vi "6AxisAccelGyro.vi"() -> ()   [LabVIEW 2024]
uses:
  Driver/Public/Digital Pull Direction.ctl
  Register.ctl
  51c12f6e-4a21-4d98-9fb3-1a2e6b8270e3.vi
  Driver/CTIPicoVISA.lvlib
panel:
  out "Waveform Chart":cluster{"[0]":dbl, "[1]":dbl, "[2]":dbl}(graph)
  out "Array":dbl[](array[numeric]) format="%.2f"
  out "loop":i32
  out "Identity":T1
  in  "Grove Connector":enum16{"I2C0", "I2C1"}(ring)
  in  "stop":bool
  in  "VISA resource name in":refnum<visa-resource-name>="COM7"
  out "error out":errorcluster
  # "https://wiki.seeedstudio.com/Grove-6-Axis_AccelerometerAndGyroscope/"
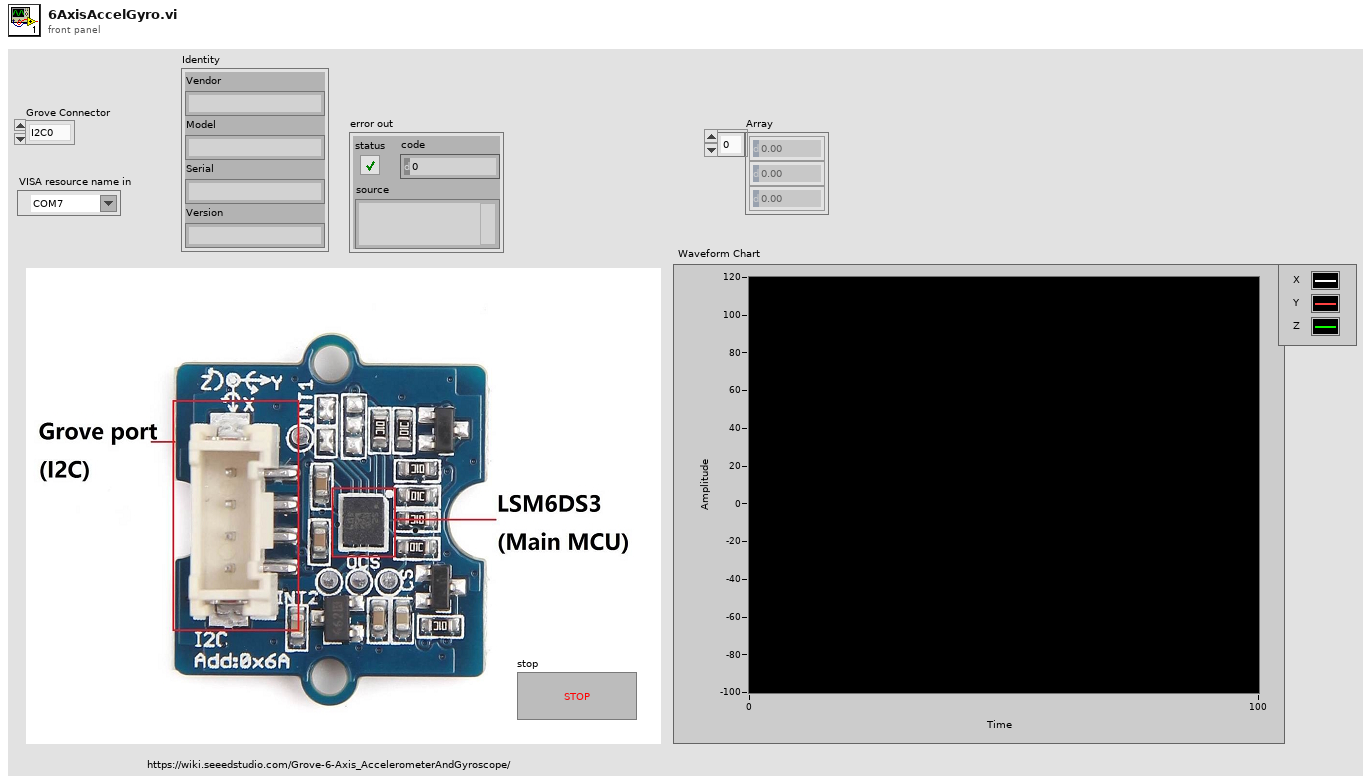
[diagram p1: front panel]
types:
  T1 = cluster{"Vendor":string, "Model":string, "Serial":string, "Version":string}
  T2 = typedef "CTIPicoVISA.lvlib/Digital Pull Direction.ctl" = enum16{"None", "Up", "Down", "Both"}
  T3 = typedef "Register.ctl" = enum16{"No Register - Error", "D6D_SRC", "STATUS_REG", "OUT_TEMP_L", "OUT_TEMP_H", "OUTX_L_G", "OUTX_H_G", "OUTY_L_G", "OUTY_H_G", "OUTZ_L_G", "OUTZ_H_G", "OUTX_L_XL", "OUTX_H_XL", "OUTY_L_XL", "OUTY_H_XL", "OUTZ_L_XL", "OUTZ_H_XL", "SENSORHUB1_REG", "SENSORHUB2_REG", "SENSORHUB3_REG", "SENSORHUB4_REG", "SENSORHUB5_REG", "SENSORHUB6_REG", "SENSORHUB7_REG", "SENSORHUB8_REG", "SENSORHUB9_REG", "SENSORHUB10_REG", "SENSORHUB11_REG", "SENSORHUB12_REG"}
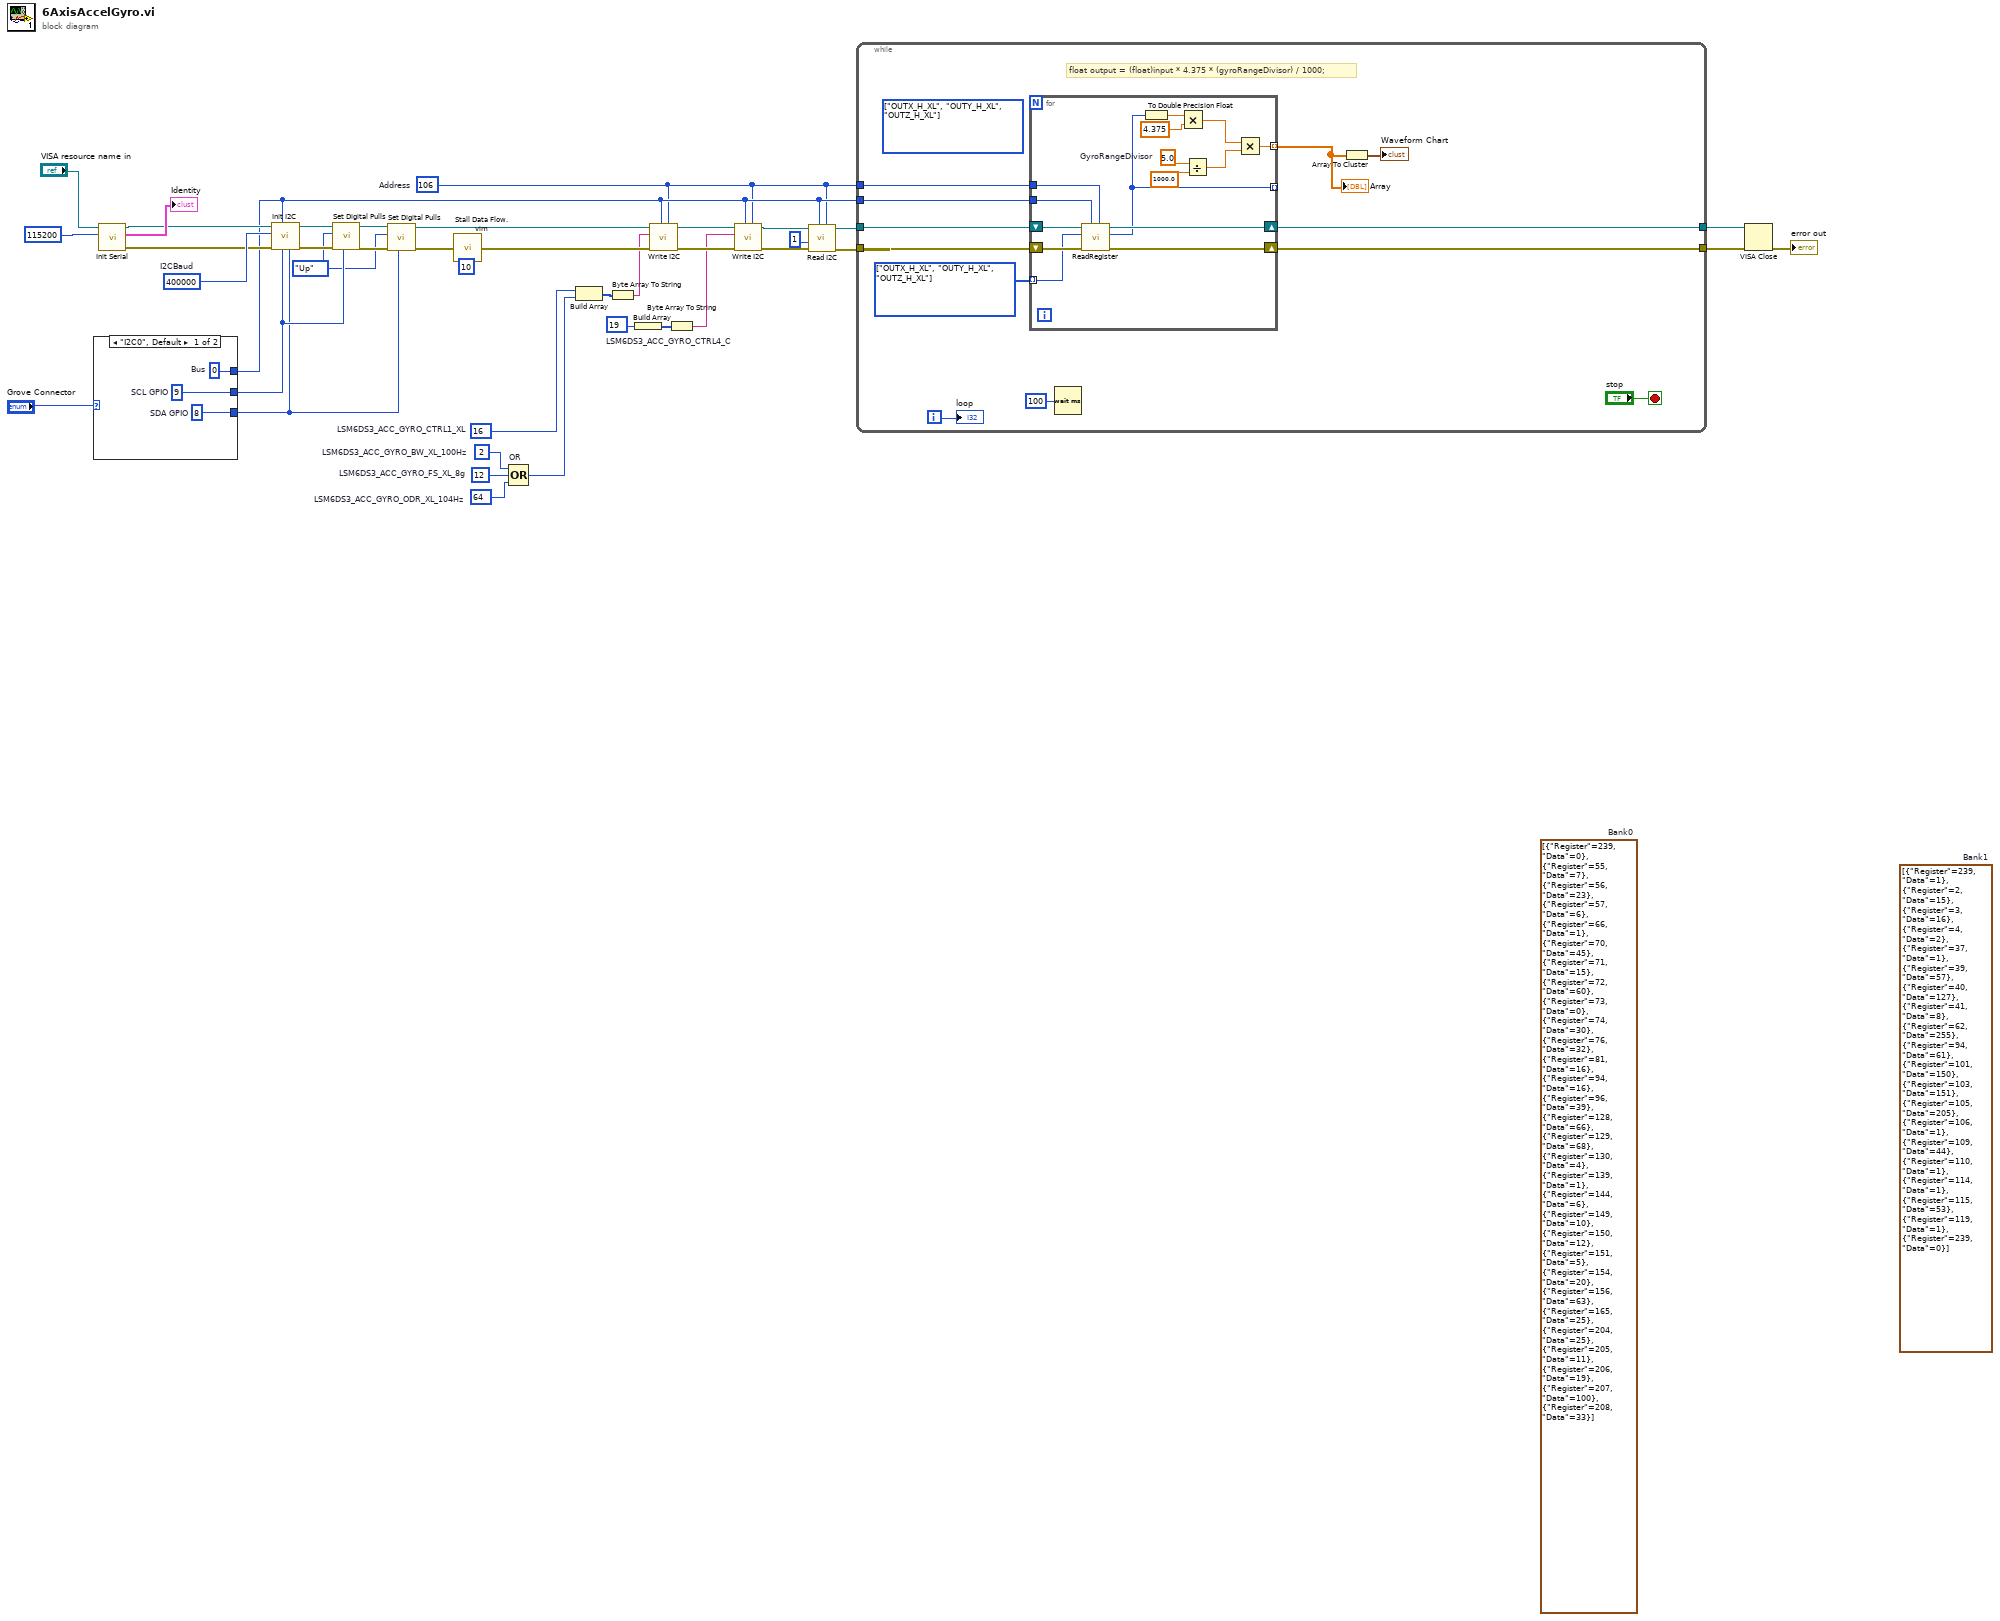
[diagram p0: block diagram]
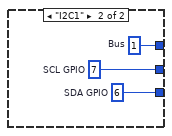
[diagram p2: hidden frame]
diagram:
  w10 = u8 19  # LSM6DS3_ACC_GYRO_CTRL4_C
  w14 = u8 64  # LSM6DS3_ACC_GYRO_ODR_XL_104Hz
  w15 = u8 12  # LSM6DS3_ACC_GYRO_FS_XL_8g
  w16 = u8 2  # LSM6DS3_ACC_GYRO_BW_XL_100Hz
  (unwired) cluster{"Register":u8, "Data":u8}[] [{"Register"=239, "Data"=0}, {"Register"=55, "Data"=7}, {"Register"=56, "Data"=23}, {"Register"=57, "Data"=6}, {"Register"=66, "Data"=1}, {"Register"=70, "Data"=45}, {"Register"=71, "Data"=15}, {"Register"=72, "Data"=60}, {"Register"=73, "Data"=0}, {"Register"=74, "Data"=30}, {"Register"=76, "Data"=32}, {"Register"=81, "Data"=16}, {"Register"=94, "Data"=16}, {"Register"=96, "Data"=39}, {"Register"=128, "Data"=66}, {"Register"=129, "Data"=68}, {"Register"=130, "Data"=4}, {"Register"=139, "Data"=1}, {"Register"=144, "Data"=6}, {"Register"=149, "Data"=10}, {"Register"=150, "Data"=12}, {"Register"=151, "Data"=5}, {"Register"=154, "Data"=20}, {"Register"=156, "Data"=63}, {"Register"=165, "Data"=25}, {"Register"=204, "Data"=25}, {"Register"=205, "Data"=11}, {"Register"=206, "Data"=19}, {"Register"=207, "Data"=100}, {"Register"=208, "Data"=33}]  # Bank0
  (unwired) cluster{"Register":u8, "Data":u8}[] [{"Register"=239, "Data"=1}, {"Register"=2, "Data"=15}, {"Register"=3, "Data"=16}, {"Register"=4, "Data"=2}, {"Register"=37, "Data"=1}, {"Register"=39, "Data"=57}, {"Register"=40, "Data"=127}, {"Register"=41, "Data"=8}, {"Register"=62, "Data"=255}, {"Register"=94, "Data"=61}, {"Register"=101, "Data"=150}, {"Register"=103, "Data"=151}, {"Register"=105, "Data"=205}, {"Register"=106, "Data"=1}, {"Register"=109, "Data"=44}, {"Register"=110, "Data"=1}, {"Register"=114, "Data"=1}, {"Register"=115, "Data"=53}, {"Register"=119, "Data"=1}, {"Register"=239, "Data"=0}]  # Bank1
  w23 = Digital_Pull_Direction."Up" ("Pull")
  w1 = u8 106  # Address
  w33 = u8 16  # LSM6DS3_ACC_GYRO_CTRL1_XL
  w37 = u32 400000  # I2CBaud
  n1 = case shown="\"I2C0\", Default" "Grove Connector" {
    tunnel: [w43 w46] -> w24
    tunnel: [w42 w45] -> w22
    tunnel: [w41 w44] -> w2
    frame "I2C0", Default {
      w41 = u8 0  # Bus
      w42 = 8  # SDA GPIO
      w43 = 9  # SCL GPIO
    }
    frame "I2C1" {
      w44 = u8 1  # Bus
      w45 = 6  # SDA GPIO
      w46 = 7  # SCL GPIO
    }
  }
  n2 = call "Init Serial.vi"("Baud (115200)"=u32 115200, "VISA resource name in"="VISA resource name in") -> ("error out"=w17:errorcluster, "Identity"=→"Identity":T1, "VISA resource name Out"=w18:refnum<visa-resource-name>)  [unwired: 7 in]
  n3 = call "Init I2C.vi"("SDA GPIO"=w22, "SCL GPIO"=w24, "Bus"=w2, "error in (no error)"=w17, "Baud"=w37, "VISA resource name in"=w18) -> ("error out"=w27:errorcluster, "VISA resource name"=w28:refnum<visa-resource-name>)  [unwired: 4 in]
  n4 = call "Set Digital Pulls.vi"("GPIO"=w24, "error in (no error)"=w27, "Pull"=w23, "VISA resource name in"=w28) -> ("error out"=w25:errorcluster, "VISA resource name"=w26:refnum<visa-resource-name>)  [unwired: 6 in]
  n5 = call "Set Digital Pulls.vi"("GPIO"=w22, "error in (no error)"=w25, "Pull"=w23, "VISA resource name in"=w26) -> ("error out"=w20:errorcluster, "VISA resource name"=w21:refnum<visa-resource-name>)  [unwired: 6 in]
  n6 = call "Stall Data Flow.vim"("value in"=w20, "milliseconds to wait"=u32 10) -> ("value out"=w32:errorcluster)  [unwired: 1 out]
  n7 = Compound Arithmetic op=OR "OR"(w16, w15, w14) -> (w13:u8)
  n8 = Build Array(w33, w13) -> (w34:u8[])
  n9 = Byte Array To String(unsigned byte array=w34) -> (string=w31:string)
  n10 = Build Array(w10) -> (w9:u8[])
  n11 = call "Write I2C.vi"("Address"=w1, "Bus"=w2, "error in (no error)"=w32, "Data"=w31, "VISA resource name in"=w21) -> ("error out"=w12:errorcluster, "VISA resource name"=w11:refnum<visa-resource-name>)  [unwired: 5 in]
  n12 = Byte Array To String(unsigned byte array=w9) -> (string=w8:string)
  n13 = call "Write I2C.vi"("Address"=w1, "Bus"=w2, "error in (no error)"=w12, "Data"=w8, "VISA resource name in"=w11) -> ("error out"=w6:errorcluster, "VISA resource name"=w7:refnum<visa-resource-name>)  [unwired: 5 in]
  n14 = call "Read I2C.vi"("Address"=w1, "Bus"=w2, "error in (no error)"=w6, "Len"=u8 1, "VISA resource name in"=w7) -> ("error out"=w3:errorcluster, "VISA resource name"=w4:refnum<visa-resource-name>)  [unwired: 4 in, 1 out]
  n15 = while {
    tunnel: w3 -> [w55]
    tunnel: [w53] -> w30
    tunnel: w4 -> [w56]
    tunnel: [w57] -> w29
    tunnel: w2 -> [w51]
    tunnel: w1 -> [w50]
    i -> [w54]
    stop <- "stop" stop-if-true
    (unwired) T3[] [enum."OUTX_H_XL", enum."OUTY_H_XL", enum."OUTZ_H_XL"] items=["No Register - Error", "D6D_SRC", "STATUS_REG", "OUT_TEMP_L", "OUT_TEMP_H", "OUTX_L_G", "OUTX_H_G", "OUTY_L_G", "OUTY_H_G", "OUTZ_L_G", "OUTZ_H_G", "OUTX_L_XL", "OUTX_H_XL", "OUTY_L_XL", "OUTY_H_XL", "OUTZ_L_XL", "OUTZ_H_XL", "SENSORHUB1_REG", "SENSORHUB2_REG", "SENSORHUB3_REG", "SENSORHUB4_REG", "SENSORHUB5_REG", "SENSORHUB6_REG", "SENSORHUB7_REG", "SENSORHUB8_REG", "SENSORHUB9_REG", "SENSORHUB10_REG", "SENSORHUB11_REG", "SENSORHUB12_REG"]
    w49 = T3[] [enum."OUTX_H_XL", enum."OUTY_H_XL", enum."OUTZ_H_XL"] items=["No Register - Error", "D6D_SRC", "STATUS_REG", "OUT_TEMP_L", "OUT_TEMP_H", "OUTX_L_G", "OUTX_H_G", "OUTY_L_G", "OUTY_H_G", "OUTZ_L_G", "OUTZ_H_G", "OUTX_L_XL", "OUTX_H_XL", "OUTY_L_XL", "OUTY_H_XL", "OUTZ_L_XL", "OUTZ_H_XL", "SENSORHUB1_REG", "SENSORHUB2_REG", "SENSORHUB3_REG", "SENSORHUB4_REG", "SENSORHUB5_REG", "SENSORHUB6_REG", "SENSORHUB7_REG", "SENSORHUB8_REG", "SENSORHUB9_REG", "SENSORHUB10_REG", "SENSORHUB11_REG", "SENSORHUB12_REG"]
    # "float output = (float)input * 4.375 * (gyroRangeDivisor) / 1000;"
    n16 = for {
      tunnel: [w66] -> _ mode=indexing
      tunnel: w51 -> [w69]
      tunnel: w50 -> [w68]
      tunnel: w49 -> [w67] mode=indexing
      shift-right: [w73] -> w57
      shift-left: w56 -> [w72]
      shift-right: [w70] -> w53
      shift-left: w55 -> [w71]
      tunnel: [w59] -> w47 mode=indexing
      w63 = 5.0  # GyroRangeDivisor
      n17 = call "ReadRegister.vi"("Address"=w68, "Bus"=w69, "error in (no error)"=w71, "Register"=w67, "VISA Refnum in"=w72) -> ("error out"=w70:errorcluster, "Numeric"=w66:i16, "VISA Refnum out"=w73:refnum<visa-resource-name>)  [unwired: 4 in]
      n18 = To Double Precision Float(number=w66) -> (double precision float=w65:dbl)
      n19 = Multiply(x=w65, y=4.375) -> (x*y=w60:dbl)
      n20 = Divide(x=w63, y=1000.0) -> (x/y=w61:dbl)
      n21 = Multiply(x=w60, y=w61) -> (x*y=w59:dbl)
    }
    "Array" <- w47
    n22 = Wait (ms)(milliseconds to wait=u32 100) -> ()  [unwired: 1 out]
    n23 = Array To Cluster(array=w47) -> (cluster=→"Waveform Chart":cluster{"[0]":dbl, "[1]":dbl, "[2]":dbl})
    "loop" <- w54
  }
  n24 = VISA Close(VISA resource name=w29, error in (no error)=w30) -> (error out=→"error out":errorcluster)
